vi "CC FITS Write Filter Names.vi"(8 "error in (no error)":errorcluster, 11 "gfits refnum":T1) -> (0 "error out":errorcluster, 3 "dup gfits refnum":T1)   [LabVIEW 2021]
uses:
  <userlib>/gfitsio/gfitsio-refnum.ctl
  Logging/CC enum Current Values Action.ctl
  <userlib>/gfitsio/gfitsio-write-key-string.vi
  hk-channel-class/HK Table/HK Table.lvclass
  <userlib>/gfitsio/gfitsio.lvlib
  Filter Wheel/Filter Wheel Object/Filter Wheel.lvclass
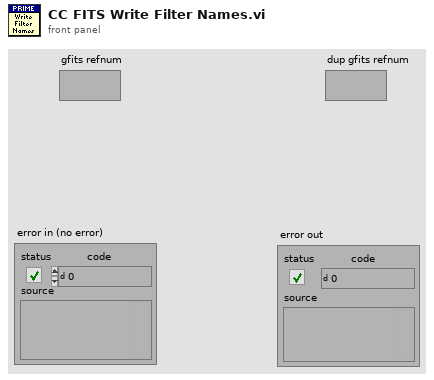
[diagram p1: front panel]
types:
  T1 = typedef "gfitsio.lvlib/gfitsio-refnum.ctl" = refnum<k1>
  T2 = typedef "CC enum Current Values Action.ctl" = enum16{"Init", "Write Item", "Write Array", "Read Item", "Read Array", "Read All", "Add Channels", "New File", "Add Message", "Get Current Values", "Close"}
  T3 = typedef "Filter Wheel.lvclass/Filter Wheel configuration.ctl" = cluster{"Num Wheels":i32, "Filters":T4[], "Invalid Combinations":i32[][], "Addr":refnum<visa-resource-name>, "Name":string, "Simulate":bool, "Homing Parameters":T5, "Default Speed":u16}
  T4 = typedef "Filter Wheel.lvclass/Filter Wheel Details.ctl" = cluster{"Names":string[], "Relative Position":i32[], "Wheel Name":string}
  T5 = typedef "Filter Wheel Arduino Homing cluster.ctl" = cluster{"Direction (F: CW)":bool, "Speed":i32, "Accel":i32, "Min Distance":i32, "Short Leg":i32, "Error Cnts":i32}
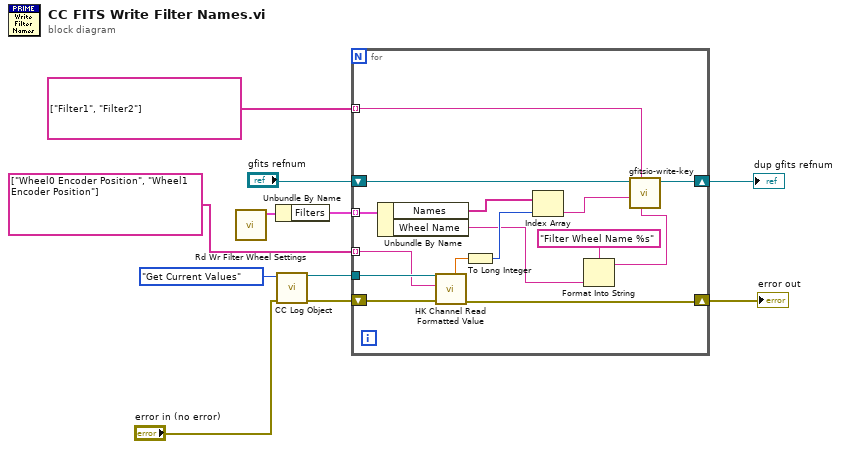
[diagram p0: block diagram]
diagram:
  n1 = call "Rd Wr Filter Wheel Settings.vi"() -> ("Filter Wheel Settings"=w3:T3)  [unwired: 10 in, 1 out]
  n2 = Unbundle By Name(w3) -> ("Filters"=w2:T4[])
  n3 = call "CC Log Object.vi"("error in (no error)"="error in (no error)", "Action"=CC_enum_Current_Values_Action."Get Current Values") -> ("error out"=w6:errorcluster, "HK Channel out"=w10:refnum<class "HK Table.lvclass">)  [unwired: 7 in, 1 out]
  n4 = for {
    tunnel: w10 -> [w26]
    shift-right: [w24] -> w8
    shift-left: "gfits refnum" -> [w25]
    shift-right: [w22] -> w5
    shift-left: w6 -> [w23]
    tunnel: string[] ["Wheel0 Encoder Position", "Wheel1 Encoder Position"] -> [w21] mode=indexing
    tunnel: w2 -> [w19] mode=indexing
    tunnel: string[] ["Filter1", "Filter2"] -> [w15] mode=indexing
    n5 = Unbundle By Name(w19) -> ("Names"=w18:string[], "Wheel Name"=w13:string)
    n6 = call-dynamic "HK Channel Read Formatted Value.vi"("error in (no error)"=w23, "Name"=w21, "HK Channel in"=w26) -> ("error out"=w22:errorcluster, "Value"=w20:dbl)  [unwired: 1 in, 6 out]
    n7 = To Long Integer(number=w20) -> (32bit integer=w17:i32)
    n8 = Index Array(array=w18, index=w17) -> (element=w16:string)
    n9 = Format Into String(format string="Filter Wheel Name %s", w13) -> (resulting string=w12:string)  [unwired: 2 in, 1 out]
    n10 = call-poly <userlib>:"gfitsio-write-key.vi"("comment"=w12, "keyname"=w15, "value"=w16, "gfits refnum"=w25) -> ("dup gfits refnum"=w24:T1)  [unwired: 6 in, 1 out]
  }
  "error out" <- w5
  "dup gfits refnum" <- w8
